vi "fg_references.vi"(7 "fg_command":T2=enum."read", 8 "error in (no error)":errorcluster, 11 "references in":T1) -> (0 "error out":errorcluster, 3 "references out":T1)   [LabVIEW 2015, in "lv-waitgroup.lvlib"]
uses:
  lv-waitgroup.lvlib
  _controls/fg_command.ctl
  _controls/references.ctl
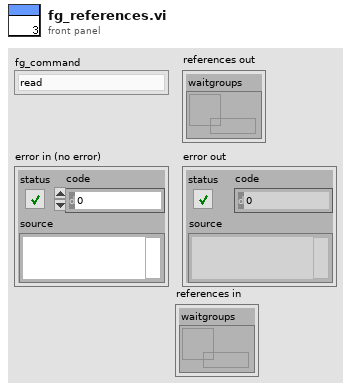
[diagram p1: front panel]
types:
  T1 = typedef "lv-waitgroup.lvlib/references.ctl" = cluster{"waitgroups":refnum<data-value>}
  T2 = typedef "lv-waitgroup.lvlib/fg_command.ctl" = enum16{"<fg_command>", "initialize", "read", "write", "shutdown", "<null>"}
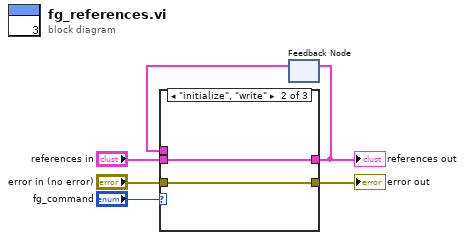
[diagram p0: block diagram]
diagram:
  n1 = feedback #1() -> (w3:T1)  [unwired: 1 in]
  n2 = case shown="\"initialize\", \"write\"" "fg_command" {
    tunnel: "error in (no error)" -> [w8 w9 w11]
    tunnel: [w8 w9 w11] -> w4
    tunnel: w3 -> [w7 _ _]
    tunnel: [w7 w10 _] -> w2
    tunnel: "references in" -> [_ w10 _]
    frame Default {
    }
    frame "initialize", "write" {
    }
    frame "shutdown" {
    }
  }
  "error out" <- w4
  "references out" <- w2
  n3 = feedback-in #1(w2) -> ()
